vi "Disable and Grey Control.vi"(0 "Control Ref":refnum<vi>[](array[refnum]), 7 "error in (no error)":errorcluster) -> (8 "error out":errorcluster)   [LabVIEW 2023, in "TLB` InstStu GPlugin Template.lvlib"]
uses:
  TLB` InstStu GPlugin Template.lvlib
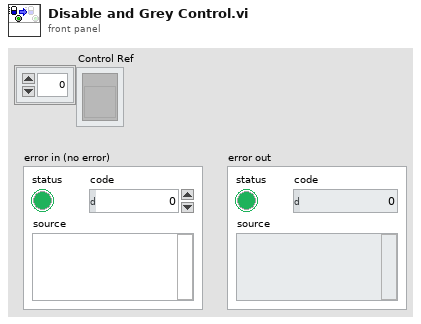
[diagram p1: front panel]
types:
  T1 = enum8{"Enabled", "Disabled", "Disabled and Grayed Out"}
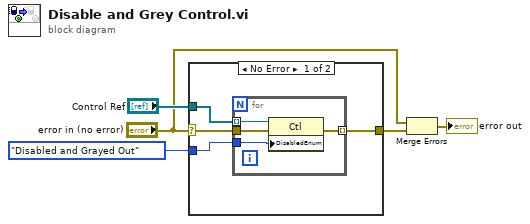
[diagram p0: block diagram]
diagram:
  n1 = case shown="No Error" "error in (no error)" {
    selector: "error in (no error)" -> [w6 _]
    tunnel: T1."Disabled and Grayed Out" ("Disabled") -> [w9 _]
    tunnel: "Control Ref" -> [w8 _]
    tunnel: [w7 _] -> w3
    frame No Error {
      n2 = for {
        tunnel: w8 -> [w13] mode=indexing
        tunnel: w9 -> [w12]
        tunnel: w6 -> [w11]
        tunnel: [w10] -> w7 mode=indexing
        n3 = property class="Ctl"(reference=w13, error in=w11, "DisabledEnum"=w12) -> (error out=w10:errorcluster)  [unwired: 1 out]
      }
    }
    frame Error {
    }
  }
  n4 = Merge Errors("error in (no error)", w3) -> (→"error out":errorcluster)
